vi "Generate Bezier Spline.vi"(8 "ending orientation":sgl=nan, 9 "starting orientation":sgl, 10 "percision":sgl=0.01, 11 "waypts":cluster{"x":sgl, "y":sgl}[](array[cluster])) -> (0 "cubic spline ctrl pts":cluster{sgl, sgl}[][](array[cluster]), 1 "Tangents":cluster{sgl, sgl}[](array[cluster]), 2 "ctrl pts":cluster{sgl, sgl}[][](array[cluster]), 3 "bezier spline":T1)   [LabVIEW 2019]
uses:
  Types/Bezier Spline.ctl
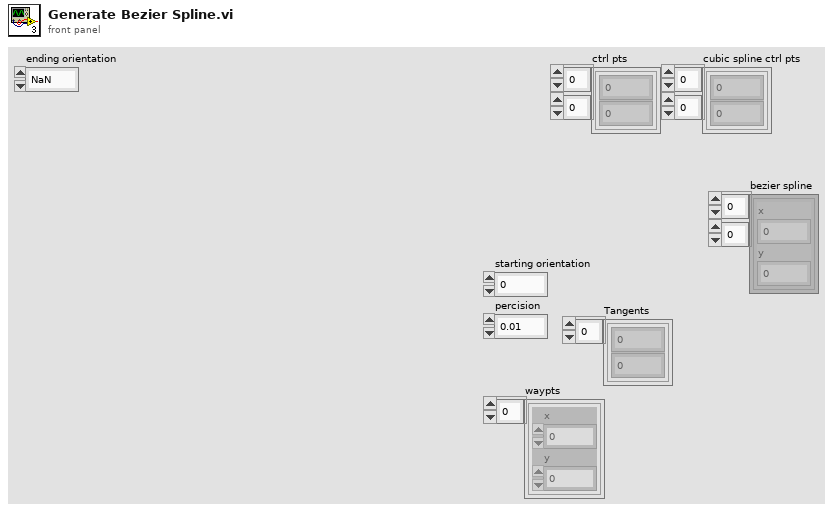
[diagram p1: front panel]
types:
  T1 = typedef "Bezier Spline.ctl" = cluster{"x":sgl, "y":sgl}[][]
  T2 = typedef "Bezier Curve.ctl" = cluster{"x":sgl, "y":sgl}[]
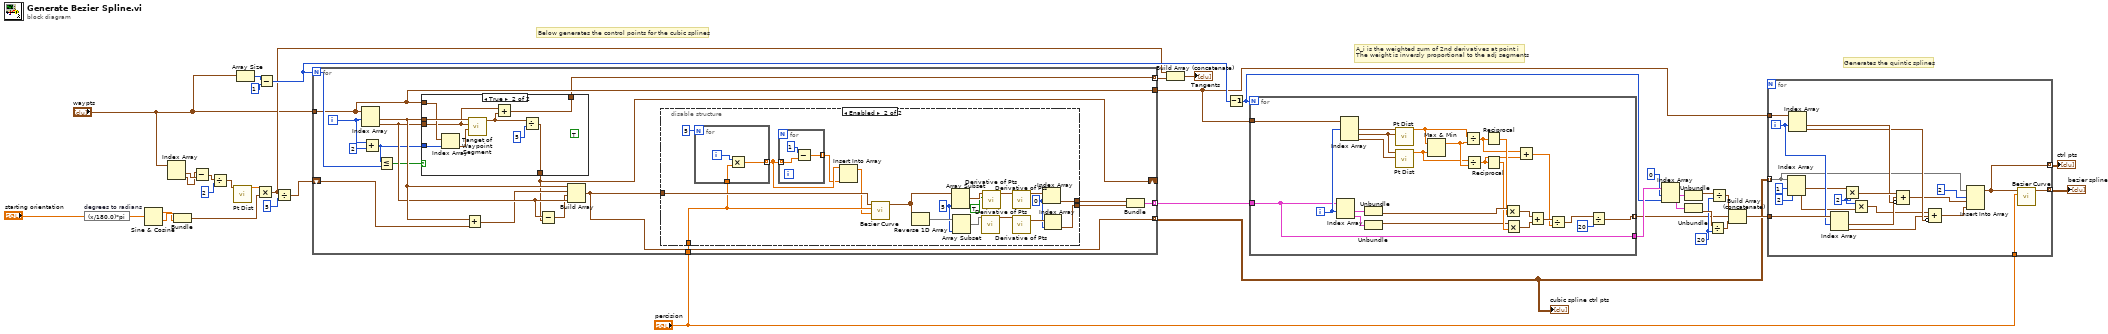
[diagram p0: block diagram]
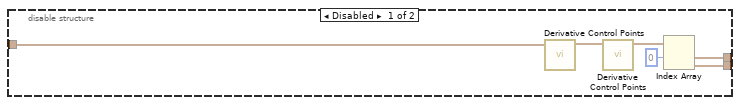
[diagram p2: hidden frame]
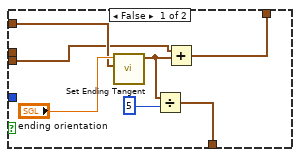
[diagram p3: hidden frame]
diagram:
  w17 = 20
  # "Generates the quintic splines"
  # "Below generates the control points for the cubic splines"
  # "A_i is the weighted sum of 2nd derivatives at point i\nThe weight is inversly proportional to the adj segments"
  n1 = expression code="(x/180.0)*pi" "degrees to radians"("starting orientation") -> (w5:sgl)
  n2 = Sine & Cosine(0:w5) -> (1:w2:sgl, 2:w3:sgl)
  n3 = Index Array(array="waypts") -> (element #1=w36:cluster{"x":sgl, "y":sgl}, element #2=w35:cluster{"x":sgl, "y":sgl})  [unwired: 2 in]
  n4 = Bundle(w3, w2) -> (w32:cluster{sgl, sgl})  [unwired: 1 in]
  n5 = Subtract(x=w35, y=w36) -> (x-y=w34:cluster{"x":sgl, "y":sgl})
  n6 = Divide(x=w34, y=u16 2) -> (x/y=w11:cluster{"x":sgl, "y":sgl})
  n7 = call "Pt Dist.vi"("point a"=w11) -> ("dist"=w12:sgl)  [unwired: 10 in]
  n8 = Array Size(array="waypts") -> (size(s)=w38:i32)
  n9 = Multiply(x=w12, y=w32) -> (x*y=w7:cluster{sgl, sgl})
  n10 = Subtract(x=w38, y=1) -> (x-y=w29:i32)
  n11 = Divide(x=w7, y=u16 5) -> (x/y=w9:cluster{sgl, sgl})
  n12 = for {
    N: w29 -> [w45]
    tunnel: "waypts" -> [w44]
    shift-right: [w43] -> _
    shift-left: w9 -> [w47]
    tunnel: [w42] -> w25 mode=indexing
    tunnel: [w50] -> w30 mode=indexing
    tunnel: [w44] -> w1
    tunnel: "percision" -> [w41]
    tunnel: [w40] -> w10 mode=indexing
    i -> [w49]
    n13 = Index Array(array=w44, index #1=w49) -> (element #1=w56:cluster{"x":sgl, "y":sgl}, element #2=w55:cluster{"x":sgl, "y":sgl})  [unwired: 1 in]
    n14 = Add(x=w49, y=2) -> (x+y=w46:i32)
    n15 = Less Or Equal?(x=w46, y=w45) -> (x <= y?=w39:bool)
    n16 = case shown="True" w39 {
      tunnel: w56 -> [_ w103]
      tunnel: w55 -> [w88 w96]
      tunnel: [w89 w101] -> w43
      tunnel: w46 -> [_ w100]
      tunnel: w44 -> [w92 w99]
      tunnel: [w90 w95] -> w40
      frame False {
        n17 = call "Set Ending Tangent.vi"("waypts"=w92, "ending orientation"="ending orientation") -> ("ending tangent"=w91:cluster{sgl, sgl})  [unwired: 9 in]
        n18 = Divide(x=w91, y=u16 5) -> (x/y=w89:cluster{sgl, sgl})
        n19 = Add(x=w88, y=w91) -> (x+y=w90:cluster{sgl, sgl})
      }
      frame True {
        (unwired) TRUE ("test")
        n20 = Index Array(array=w99, index=w100) -> (element=w98:cluster{"x":sgl, "y":sgl})
        n21 = call "Tanget of Waypoint Segment.vi"("point c"=w98, "point b"=w96, "point a"=w103) -> ("T_i"=w97:cluster{sgl, sgl})  [unwired: 8 in]
        n22 = Add(x=w96, y=w97) -> (x+y=w95:cluster{sgl, sgl})
        n23 = Divide(x=w97, y=u16 5) -> (x/y=w101:cluster{sgl, sgl})
      }
    }
    n24 = Add(x=w56, y=w47) -> (x+y=w54:cluster{sgl, sgl})
    n25 = Subtract(x=w55, y=w43) -> (x-y=w53:cluster{sgl, sgl})
    n26 = Build Array(w56, w54, w53, w55) -> (w42:cluster{"x":sgl, "y":sgl}[])
    n27 = disable-structure shown="Enabled" {
      disable-tunnel: w42 -> [w61 w69]
      disable-tunnel: [w58 w72] -> w52
      disable-tunnel: [w57 w71] -> w51
      disable-tunnel: w41 -> [_ w67]
      frame Disabled {
        n28 = call "Derivative Control Points.vi"("ctrl points"=w61) -> ("d ctrl pts"=w62:cluster{dbl, dbl}[])  [unwired: 10 in]
        n29 = call "Derivative Control Points.vi"("ctrl points"=w62) -> ("d ctrl pts"=w60:cluster{dbl, dbl}[])  [unwired: 10 in]
        n30 = Index Array(array=w60, index #1=0 ("index")) -> (element #1=w58:cluster{dbl, dbl}, element #2=w57:cluster{dbl, dbl})  [unwired: 1 in]
      }
      frame Enabled {
        w74 = 0 ("index")
        w73 = 5 ("length")
        n31 = for {
          N: 5 -> [_]
          tunnel: w67 -> [w86]
          tunnel: [w85] -> w64 mode=indexing
          i -> [w87]
          n32 = Multiply(x=w87, y=w86) -> (x*y=w85:sgl)
        }
        n33 = for {
          tunnel: w64 -> [w84] mode=indexing
          tunnel: [w82] -> w63 mode=indexing
          n34 = Subtract(x=1 ("length"), y=w84) -> (x-y=w82:sgl)
        }
        n35 = Insert Into Array(array=w64, new element=w63) -> (w66:sgl[])  [unwired: 1 in]
        n36 = call "Bezier Curve.vi"("position"=w66, "percision"=w67, "ctrl points"=w69) -> ("curve"=w65:T2)  [unwired: 8 in]
        n37 = Reverse 1D Array(array=w65) -> (reversed array=w81:T2)
        n38 = Array Subset(array=w65, length=w73) -> (w80:T2)  [unwired: 1 in]
        n39 = Array Subset(array=w81, length=w73) -> (w78:T2)  [unwired: 1 in]
        n40 = call "Derivative of Pts.vi"("pts"=w78) -> ("pts out"=w77:cluster{sgl, sgl}[])  [unwired: 10 in]
        n41 = call "Derivative of Pts.vi"("fix first pt?"=TRUE, "pts"=w80) -> ("pts out"=w79:cluster{sgl, sgl}[])  [unwired: 9 in]
        n42 = call "Derivative of Pts.vi"("pts"=w79) -> ("pts out"=w76:cluster{sgl, sgl}[])  [unwired: 10 in]
        n43 = call "Derivative of Pts.vi"("pts"=w77) -> ("pts out"=w75:cluster{sgl, sgl}[])  [unwired: 10 in]
        n44 = Index Array(array=w76, index=w74) -> (element=w72:cluster{sgl, sgl})
        n45 = Index Array(array=w75, index=w74) -> (element=w71:cluster{sgl, sgl})
      }
    }
    n46 = Bundle(w52, w51) -> (w50:cluster{cluster{sgl, sgl}, cluster{sgl, sgl}})  [unwired: 1 in]
  }
  "cubic spline ctrl pts" <- w25
  n47 = Build Array (concatenate)(w7, w10) -> (→"Tangents":cluster{sgl, sgl}[])
  n48 = Decrement(x=w29) -> (x-1=w22:i32)
  n49 = for {
    N: w22 -> [_]
    tunnel: w30 -> [w118]
    tunnel: w1 -> [w117]
    tunnel: [w107] -> w13 mode=indexing
    tunnel: [w118] -> w28
    i -> [w127]
    n50 = Index Array(array=w118, index #1=w127) -> (element #1=w126:cluster{cluster{sgl, sgl}, cluster{sgl, sgl}}, element #2=w125:cluster{cluster{sgl, sgl}, cluster{sgl, sgl}})  [unwired: 1 in]
    n51 = Index Array(array=w117, index #1=w127) -> (element #1=w124:cluster{"x":sgl, "y":sgl}, element #2=w123:cluster{"x":sgl, "y":sgl}, element #3=w122:cluster{"x":sgl, "y":sgl})  [unwired: 2 in]
    n52 = Unbundle(w126) -> (w115:cluster{sgl, sgl})  [unwired: 1 out]
    n53 = Unbundle(w125) -> (w112:cluster{sgl, sgl})  [unwired: 1 out]
    n54 = call "Pt Dist.vi"("point b"=w123, "point a"=w124) -> ("dist"=w121:sgl)  [unwired: 9 in]
    n55 = call "Pt Dist.vi"("point b"=w122, "point a"=w123) -> ("dist"=w119:sgl)  [unwired: 9 in]
    n56 = Max & Min(x=w121, y=w119) -> (max(x,y)=w120:sgl)  [unwired: 1 out]
    n57 = Divide(x=w121, y=w120) -> (x/y=w106:sgl)
    n58 = Divide(x=w119, y=w120) -> (x/y=w105:sgl)
    n59 = Reciprocal(x=w106) -> (1/x=w114:sgl)
    n60 = Reciprocal(x=w105) -> (1/x=w113:sgl)
    n61 = Multiply(x=w115, y=w114) -> (x*y=w111:cluster{sgl, sgl})
    n62 = Multiply(x=w112, y=w113) -> (x*y=w110:cluster{sgl, sgl})
    n63 = Add(x=w106, y=w105) -> (x+y=w104:sgl)
    n64 = Add(x=w111, y=w110) -> (x+y=w109:cluster{sgl, sgl})
    n65 = Divide(x=w109, y=w104) -> (x/y=w108:cluster{sgl, sgl})
    n66 = Divide(x=w108, y=20) -> (x/y=w107:cluster{sgl, sgl})
  }
  n67 = Index Array(array=w28, index #1=0 ("index"), index #2=w22) -> (element #1=w27:cluster{cluster{sgl, sgl}, cluster{sgl, sgl}}, element #2=w24:cluster{cluster{sgl, sgl}, cluster{sgl, sgl}})
  n68 = Unbundle(w27) -> (w18:cluster{sgl, sgl})  [unwired: 1 out]
  n69 = Unbundle(w24) -> (w20:cluster{sgl, sgl})  [unwired: 1 out]
  n70 = Divide(x=w20, y=w17) -> (x/y=w19:cluster{sgl, sgl})
  n71 = Divide(x=w18, y=w17) -> (x/y=w16:cluster{sgl, sgl})
  n72 = Build Array (concatenate)(w16, w13, w19) -> (w26:cluster{sgl, sgl}[])
  n73 = for {
    tunnel: w26 -> [w145]
    tunnel: w25 -> [w134] mode=indexing
    tunnel: w1 -> [w146]
    tunnel: "percision" -> [w130]
    tunnel: [w129] -> w21 mode=indexing
    tunnel: [w128] -> w15 mode=indexing
    i -> [w144]
    w141 = u16 2
    n74 = Index Array(array=w134, index #1=1 ("index"), index #2=2 ("index")) -> (element #1=w143:cluster{"x":sgl, "y":sgl}, element #2=w142:cluster{"x":sgl, "y":sgl})
    n75 = Index Array(array=w146, index #1=w144) -> (element #1=w138:cluster{"x":sgl, "y":sgl}, element #2=w137:cluster{"x":sgl, "y":sgl})  [unwired: 1 in]
    n76 = Index Array(array=w145, index #1=w144) -> (element #1=w139:cluster{sgl, sgl}, element #2=w135:cluster{sgl, sgl})  [unwired: 1 in]
    n77 = Multiply(x=w143, y=w141) -> (x*y=w140:cluster{"x":sgl, "y":sgl})
    n78 = Multiply(x=w141, y=w142) -> (x*y=w136:cluster{"x":sgl, "y":sgl})
    n79 = Compound Arithmetic op=ADD(w140, w139, invert w138) -> (w133:cluster{sgl, sgl})
    n80 = Compound Arithmetic op=ADD(w136, w135, invert w137) -> (w132:cluster{sgl, sgl})
    n81 = Insert Into Array(array=w134, index=2, new element #1=w133, new element #2=w132) -> (w128:cluster{"x":sgl, "y":sgl}[])
    n82 = call "Bezier Curve.vi"("percision"=w130, "ctrl points"=w128) -> ("curve"=w129:T2)  [unwired: 9 in]
  }
  "bezier spline" <- w21
  "ctrl pts" <- w15
